vi "FichierExiste.vi"(3 "entrée d'erreur (pas d'erreur)":errorcluster, 5 "cheminProchainFichierRAW":path) -> (0 "sortie d'erreur":errorcluster, 1 "Booléen":bool, 2 "path out":path)   [LabVIEW 2017]
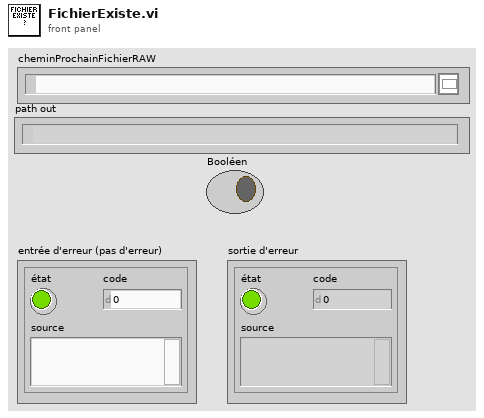
[diagram p1: front panel]
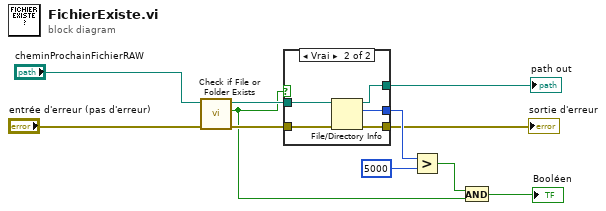
[diagram p0: block diagram]
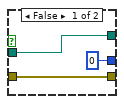
[diagram p2: hidden frame]
diagram:
  n1 = call <vilib>:"Check if File or Folder Exists.vi"("error in (no error)"="entrée d'erreur (pas d'erreur)", "path"="cheminProchainFichierRAW") -> ("error out"=w4:errorcluster, "file or folder exists?"=w1:bool, "dup path"=w8:path)  [unwired: 7 in]
  n2 = case shown="Vrai" w1 {
    tunnel: [i64 0 ("size") w19] -> w10
    tunnel: [w14 w18] -> w9
    tunnel: w8 -> [w14 w17]
    tunnel: [w13 w16] -> w5
    tunnel: w4 -> [w13 w15]
    frame False {
    }
    frame True {
      n3 = File/Directory Info(path=w17, error in=w15) -> (path out=w18:path, size=w19:i64, error out=w16:errorcluster)  [unwired: 4 out]
    }
  }
  "path out" <- w9
  "sortie d'erreur" <- w5
  n4 = Greater?(x=w10, y=i64 5000) -> (0:w6:bool)
  n5 = And(x=w6, y=w1) -> (x .and. y?=→"Booléen":bool)
